vi "VisionAim.vi"(8 "Reset PID":bool, 11 "Angle":dbl) -> (2 "In Range":bool, 3 "Turn":dbl)   [LabVIEW 2020]
doc: "Uses PID to output turn amount to turn robot towards target"
uses:
  Framework/Robot Global Data.vi
panel:
  in  "Latency":i32=7
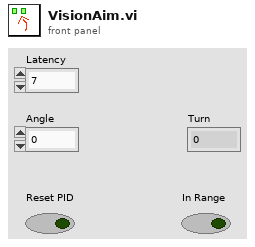
[diagram p1: front panel]
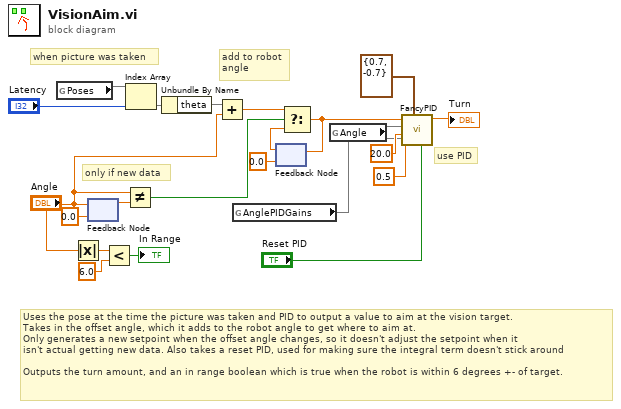
[diagram p0: block diagram]
diagram:
  # "add to robot\nangle"
  # "use PID"
  # "only if new data"
  # "when picture was taken"
  # "Uses the pose at the time the picture was taken and PID to output a value to aim at the vision target.\nTakes in the offset angle, which it adds to the robot angle to get where to aim at.\nOnly generates a new setpoint when the offset angle changes, so it doesn't adjust the setpoint when it\nisn't actual getting new data. Also takes a reset PID, used for making sure the integral term doesn't stick around\n\nOutputs the turn amount, and an in range boolean which is true when the robot is within 6 degrees +- of target."
  n1 = global read "Robot Global Data.vi" "Poses"() -> (w22)
  n2 = Absolute Value(x="Angle") -> (abs(x)=w18:dbl)
  n3 = feedback-in #1("Angle") -> ()
  n4 = feedback #1(0.0 ("Angle")) -> (w19:dbl)
  n5 = Less?(x=w18, y=6.0) -> (x < y?=→"In Range":bool)
  n6 = Not Equal?(x="Angle", y=w19) -> (x != y?=w9:bool)
  n7 = Index Array(array=w22, index="Latency") -> (element=w15)
  n8 = Unbundle By Name(w15) -> ("theta"=w14)
  n9 = Add(x=w14, y="Angle") -> (x+y=w12:dbl)
  n10 = global read "Robot Global Data.vi" "AnglePIDGains"() -> (w1)
  n11 = feedback #2(0.0 ("Angle")) -> (w10:dbl)
  n12 = Select(t=w12, s=w9, f=w10) -> (s? t:f=w2:dbl)
  n13 = feedback-in #2(w2) -> ()
  n14 = global read "Robot Global Data.vi" "Angle"() -> (w8)
  n15 = call "FancyPID.vi"("Reset"="Reset PID", "Gains"=w1, "Range"=cluster{"output high":dbl, "output low":dbl} {"output high"=0.7, "output low"=-0.7}, "Disable Range"=0.5, "Integral Range"=20.0, "Process variable"=w8, "Setpoint"=w2) -> ("output"=→"Turn":dbl)  [unwired: 4 in]
